vi "_054.vi"() -> ()   [LabVIEW 2024]
panel:
  in  "text":string
  out "error out":errorcluster
  in  "Path":path
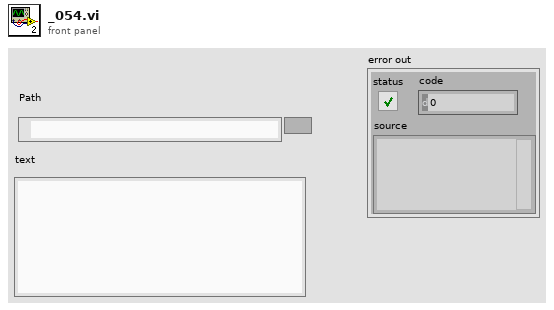
[diagram p1: front panel]
types:
  T1 = enum16{"open", "replace", "create", "open or create", "replace or create", "replace or create with confirmation"}
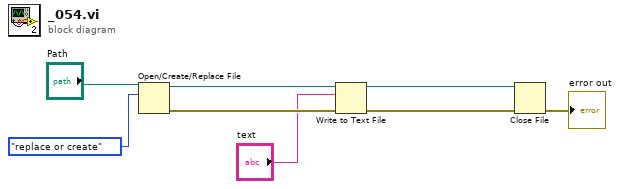
[diagram p0: block diagram]
diagram:
  n1 = Open/Create/Replace File(file path (use dialog)="Path", operation (0:open)=T1."replace or create") -> (refnum out=w8:refnum<file>, error out=w6:errorcluster)  [unwired: 4 in, 1 out]
  n2 = Write to Text File(file (use dialog)=w8, text="text", error in=w6) -> (refnum out=w7:refnum<file>, error out=w5:errorcluster)  [unwired: 1 in, 1 out]
  n3 = Close File(refnum=w7, error in=w5) -> (error out=→"error out":errorcluster)  [unwired: 1 out]
